vi "Write Touchstone File.vi"(5 "Note":string, 6 "(De-)Embed":T1(array[cluster])=[{"enabled"=FALSE, "De-embed"=TRUE, "Swap Ports Left"=FALSE, "De-embedding file"=path ""}, {"enabled"=FALSE, "De-embed"=TRUE, "Swap Ports Left"=FALSE, "De-embedding file"=path ""}], 7 "File Path":path, 8 "Error In":errorcluster, 9 "MDIF-format":bool, 10 "Parameters":cluster{"Name":string, "Value":string}[](array[cluster]), 11 "Sparameters":T2[](array[typedef]) {"Frequency" format="%#_6p"}) -> (0 "Error Out":errorcluster)   [LabVIEW 2020]
doc: "Vi for writing S2P Files.\nIt will give an error if the file is already created."
uses:
  Instruments/Vector Network Analyzer/Controls/Sparameter cluster.ctl
  <vilib>/Utility/error.llb/whitespace.ctl
  Instruments/Vector Network Analyzer/Vector Network Analyzer.lvclass
panel:
  out "Slide":u8(slide) scale=0.0..100.0
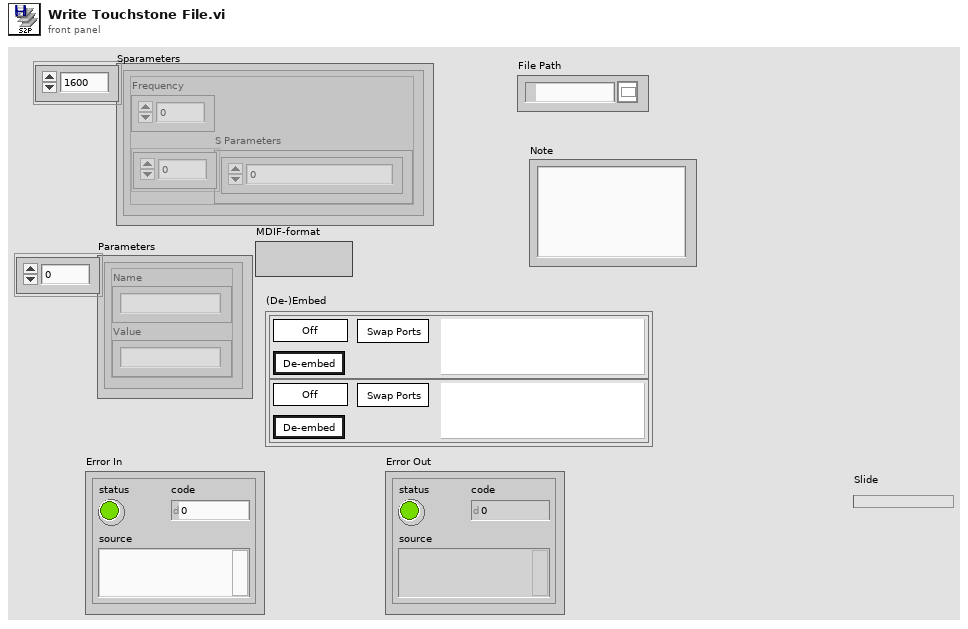
[diagram p1: front panel]
types:
  T1 = cluster{"enabled":bool, "De-embed":bool, "Swap Ports Left":bool, "De-embedding file":path}[]
  T2 = typedef "Vector Network Analyzer.lvclass/Sparameter cluster.ctl" = cluster{"Frequency":dbl, "S Parameters":cdb[]}
  T3 = cluster{"(De-)embedding file":path, "S-parameters":cdb[][], "Frequencies (Hz)":dbl[], "output string":string, "Use":bool, "Swap Ports":bool, "De-embed":bool}
  T4 = typedef "whitespace.ctl" = u16
  T5 = cluster{"enabled":bool, "De-embed":bool, "Swap Ports Left":bool, "De-embedding file":path}
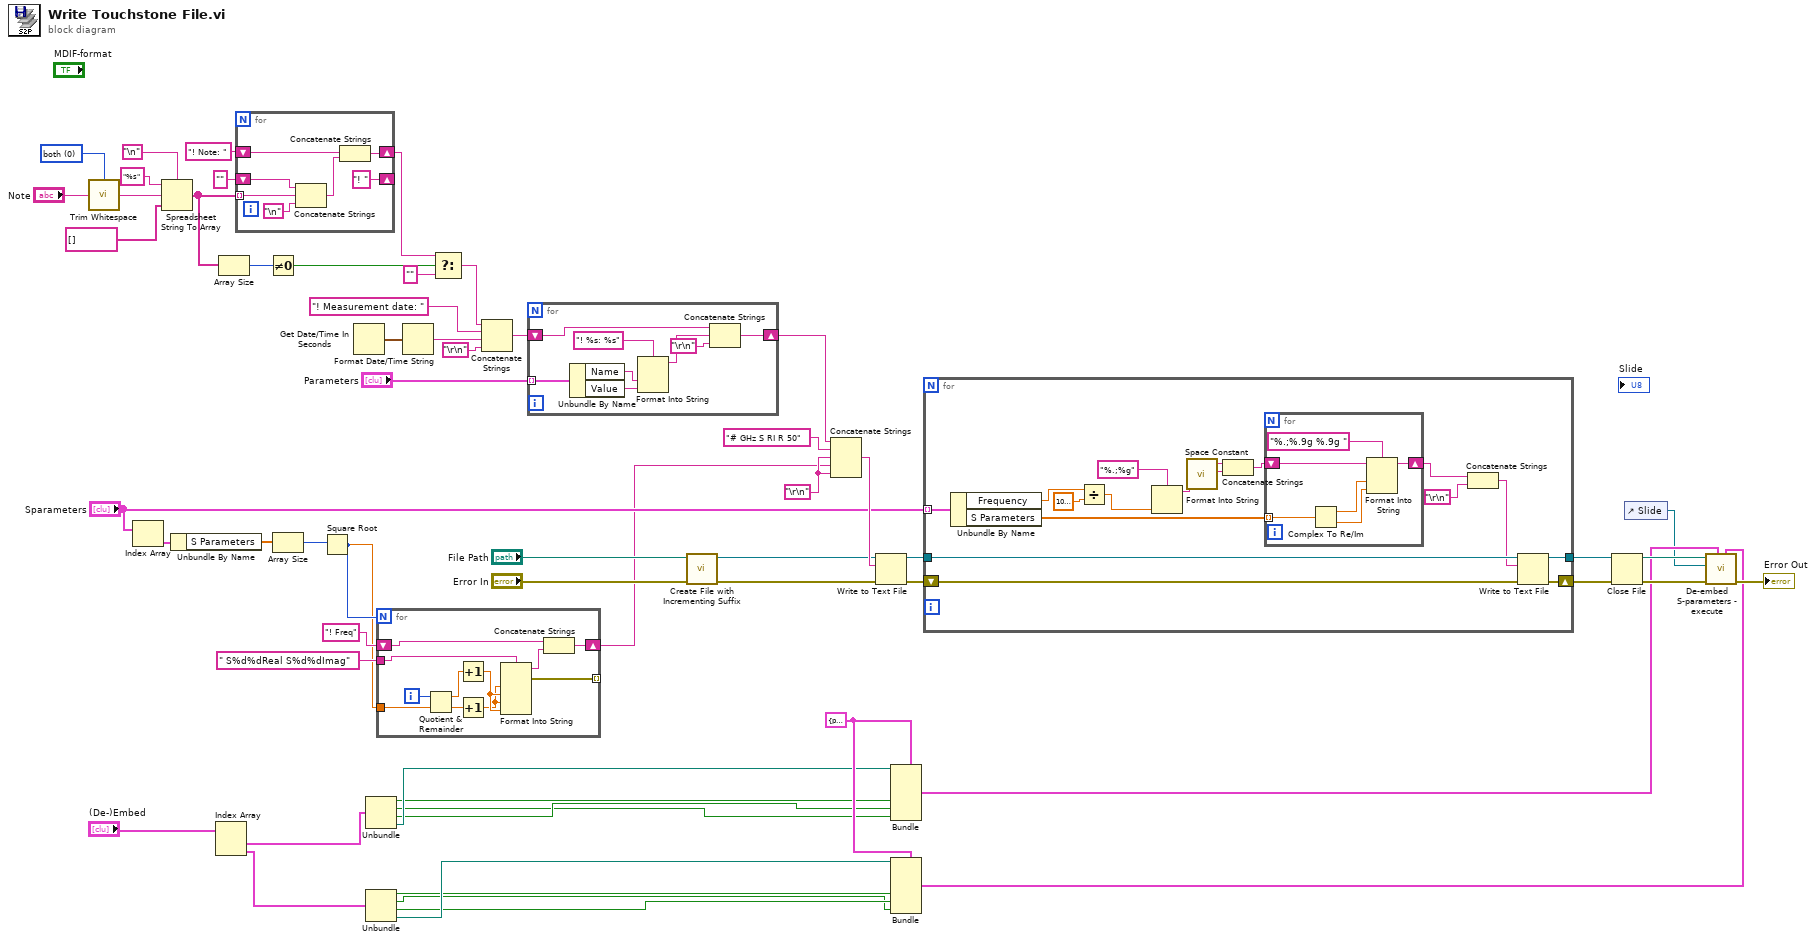
[diagram p0: block diagram]
diagram:
  w15 = T3 {"(De-)embedding file"=path "", "S-parameters"=[], "Frequencies (Hz)"=[], "output string"="", "Use"=FALSE, "Swap Ports"=FALSE, "De-embed"=FALSE} ("output cluster 2")
  w33 = T4 0 items=["both", "start of string", "end of string"] ("location (both)")
  w41 = "\r\n"
  n1 = call <vilib>:"Trim Whitespace.vi"("string"="Note", "location (both)"=w33) -> ("trimmed string"=w35:string)
  n2 = Index Array(array="Sparameters") -> (element=w25:T2)  [unwired: 1 in]
  n3 = Spreadsheet String To Array(delimiter (Tab)="\n", format string="%s", spreadsheet string=w35, array type (2D Dbl)=string[] []) -> (array=w32:string[])
  n4 = Unbundle By Name(w25) -> ("S Parameters"=w24:cdb[])
  n5 = Index Array(array="(De-)Embed") -> (element #1=w17:T5, element #2=w16:T5)  [unwired: 2 in]
  n6 = Array Size(array=w32) -> (size(s)=w31:i32)
  n7 = for {
    tunnel: w32 -> [w63] mode=indexing
    shift-right: [w64] -> w29
    shift-left: "! Note: " -> [w65]
    shift-right: ["! " ("string")] -> _
    shift-left: "" ("string") -> [w60]
    n8 = Concatenate Strings(w60, w63, "\n") -> (w62:string)
    n9 = Concatenate Strings(w65, w62) -> (w64:string)
  }
  n10 = Not Equal To 0?(x=w31) -> (x != 0?=w30:bool)
  n11 = Array Size(array=w24) -> (size(s)=w21:i32)
  n12 = Square Root(x=w21) -> (sqrt(x)=w20:dbl)
  n13 = Get Date/Time In Seconds() -> (seconds since 1Jan1904=w57:timestamp)
  n14 = Unbundle(w17) -> ("enabled"=w12:bool, "De-embed"=w8:bool, "Swap Ports Left"=w9:bool, "De-embedding file"=w13:path)
  n15 = Unbundle(w16) -> ("enabled"=w11:bool, "De-embed"=w7:bool, "Swap Ports Left"=w10:bool, "De-embedding file"=w14:path)
  n16 = for {
    N: w21 -> [_]
    tunnel: " S%d%dReal S%d%dImag" ("string") -> [w76]
    tunnel: w20 -> [w75]
    tunnel: [w73] -> _ mode=indexing
    shift-right: [w70] -> w19
    shift-left: "! Freq" ("string") -> [w72]
    i -> [w74]
    n17 = Quotient & Remainder(x=w74, y=w75) -> (x-y*floor(x/y)=w68:dbl, floor(x/y)=w69:dbl)
    n18 = Increment(x=w68) -> (x+1=w67:dbl)
    n19 = Increment(x=w69) -> (x+1=w66:dbl)
    n20 = Format Into String(format string=w76, w66, w67, w66, w67) -> (resulting string=w71:string, error out=w73:errorcluster)  [unwired: 2 in]
    n21 = Concatenate Strings(w72, w71) -> (w70:string)
  }
  n22 = Format Date/Time String(seconds (now)=w57) -> (date/time string=w55:string)  [unwired: 2 in]
  n23 = Select(t=w29, s=w30, f="") -> (s? t:f=w28:string)
  n24 = Concatenate Strings(w28, "! Measurement date: ", w55, "\r\n") -> (w53:string)
  n25 = for {
    shift-right: [w83] -> w52
    shift-left: w53 -> [w84]
    tunnel: "Parameters" -> [w82] mode=indexing
    n26 = Unbundle By Name(w82) -> ("Name"=w78:string, "Value"=w77:string)
    n27 = Format Into String(format string="! %s: %s", w78, w77) -> (resulting string=w80:string)  [unwired: 2 in, 1 out]
    n28 = Concatenate Strings(w84, w80, "\r\n") -> (w83:string)
  }
  n29 = call <vilib>:"Create File with Incrementing Suffix.vi"("error in (no error)"="Error In", "file path"="File Path") -> ("error out"=w37:errorcluster, "refnum out"=w38:refnum<file>)  [unwired: 7 in, 1 out]
  n30 = Concatenate Strings(w52, "# GHz S RI R 50", w41, w19, w41) -> (w44:string)
  n31 = Write to Text File(file (use dialog)=w38, text=w44, error in=w37) -> (refnum out=w45:refnum<file>, error out=w46:errorcluster)  [unwired: 1 in, 1 out]
  n32 = Bundle(cluster=w15, "(De-)embedding file"=w13, "Use"=w12, "Swap Ports"=w9, "De-embed"=w8) -> (w2:T3)  [unwired: 3 in]
  n33 = Bundle(cluster=w15, "(De-)embedding file"=w14, "Use"=w11, "Swap Ports"=w10, "De-embed"=w7) -> (w3:T3)  [unwired: 3 in]
  n34 = for {
    tunnel: "Sparameters" -> [w100] mode=indexing
    shift-right: [w91] -> w43
    shift-left: w46 -> [w90]
    tunnel: w45 -> [w89]
    tunnel: [w88] -> w42
    n35 = Unbundle By Name(w100) -> ("Frequency"=w96:dbl, "S Parameters"=w99:cdb[])
    n36 = Divide(x=w96, y=1000000000.0) -> (x/y=w95:dbl)
    n37 = Format Into String(format string="%.;%g", w95) -> (resulting string=w98:string)  [unwired: 2 in, 1 out]
    n38 = call <vilib>:"Space Constant.vi"() -> ("String"=w93:string)
    n39 = Concatenate Strings(w98, w93) -> (w92:string)
    n40 = for {
      tunnel: w99 -> [w102] mode=indexing
      shift-right: [w101] -> w86
      shift-left: w92 -> [w106]
      n41 = Complex To Re/Im(x + iy=w102) -> (x=w104:dbl, y=w103:dbl)
      n42 = Format Into String(format string="%.;%.9g %.9g ", initial string=w106, w104, w103) -> (resulting string=w101:string)  [unwired: 1 in, 1 out]
    }
    n43 = Concatenate Strings(w86, "\r\n") -> (w85:string)
    n44 = Write to Text File(file (use dialog)=w89, text=w85, error in=w90) -> (refnum out=w88:refnum<file>, error out=w91:errorcluster)  [unwired: 1 in, 1 out]
  }
  n45 = Close File(refnum=w42, error in=w43) -> (path=w4:path, error out=w6:errorcluster)
  n46 = control-ref of="Slide"() -> (w1:refnum<vi>)
  n47 = call "De-embed S-parameters - execute.vi"("Right info"=w3, "Left info"=w2, "error in (no error)"=w6, "Horizontal Progress Bar"=w1, "DUT+Fixture"=w4) -> ("error out"=→"Error Out":errorcluster)  [unwired: 6 in]
